vi "AVQ8347 Data Separator Select Data.vi"(8 "Error In":errorcluster, 11 "VISA Session":refnum<visa-resource-name>) -> (0 "Error Out":errorcluster, 1 "Data Separrator Select Value":u16, 2 "Return All Data":string, 3 "Copy VISA Session":refnum<visa-resource-name>)   [LabVIEW 2021]
doc: "This function returns the data separator select value"
panel:
  # "Data Separrator Select Data"
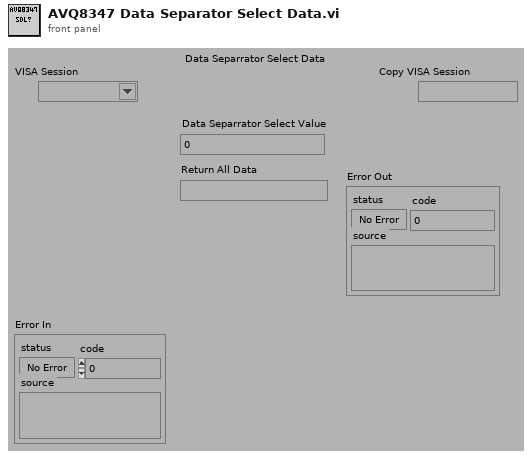
[diagram p1: front panel]
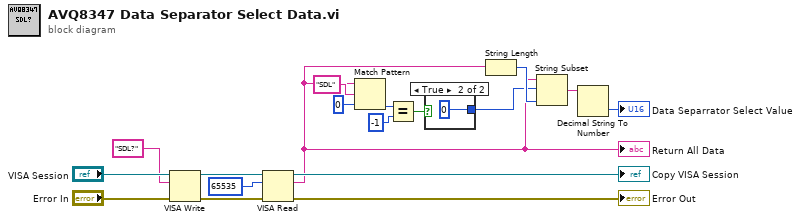
[diagram p0: block diagram]
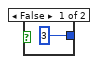
[diagram p2: hidden frame]
diagram:
  n1 = VISA Write(VISA resource name="VISA Session", write buffer="SDL?", error in (no error)="Error In") -> (VISA resource name out=w14:refnum<visa-resource-name>, error out=w13:errorcluster)  [unwired: 1 out]
  n2 = VISA Read(VISA resource name=w14, byte count=65535, error in (no error)=w13) -> (VISA resource name out=→"Copy VISA Session":refnum<visa-resource-name>, read buffer=w2:string, error out=→"Error Out":errorcluster)  [unwired: 1 out]
  "Return All Data" <- w2
  n3 = Match Pattern(string=w2, regular expression="SDL", offset (0)=0) -> (offset past match=w3:i32)  [unwired: 3 out]
  n4 = Equal?(x=w3, y=-1) -> (x = y?=w5:bool)
  n5 = case shown="True" w5 {
    tunnel: [3 0] -> w1
    frame False {
    }
    frame True {
    }
  }
  n6 = String Length(string=w2) -> (length=w15:i32)
  n7 = String Subset(string=w2, offset (0)=w1, length (rest)=w15) -> (substring=w9:string)
  n8 = Decimal String To Number(string=w9) -> (number=→"Data Separrator Select Value":i32)  [unwired: 2 in, 1 out]
